vi "Launch Controller Actor.vi"(11 "RDS Root Actor in":refnum<class "RDS Root Actor.lvclass">) -> (3 "RDS Root Actor out":refnum<class "RDS Root Actor.lvclass">)   [LabVIEW 2015, in "RDS Root Actor.lvlib" / "RDS Root Actor.lvclass"]
uses:
  RDS Root Actor.lvclass
  Libraries/RDS Framework/RDS Message ID.ctl
  RDS Controller Actor/RDS Controller Actor/RDS Controller Actor/RDS Controller Actor.lvclass
  RDS Parent Actor/RDS Parent Actor/RDS Parent Actor.lvclass/RDS Parent Actor.ctl
  RDS Parent Actor/RDS Parent Actor/RDS Parent Actor.lvclass
  Libraries/RDS Child Messages/RDS Child Messages.lvlib
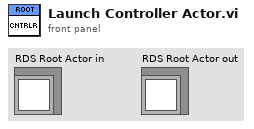
[diagram p1: front panel]
types:
  T1 = typedef "RDS Child Messages.lvlib/RDS Message ID.ctl" = enum16{"RDS Hello World", "String Message", "AIP_Status", "AIP_Command", "GPS_Data", "MCB_Command", "MCB_Status", "Compass_Data", "Depth_Data", "Battery_Data", "Contoller_State", "Set_Mag_Dev", "BTB_Shutdown", "State_Sample_Request", "State_Sample", "PID_Gains_Set", "Helm_Limiter_Set", "Helm_Heading_Command", "Helm_Steering_Command", "Helm_Status", "Controller_Message", "AIP_Set_Min_Depth", "Mission_Controller_State", "Mission_Upload", "Mission_Set_Op_and_Run", "Mission_Settings_Set"}
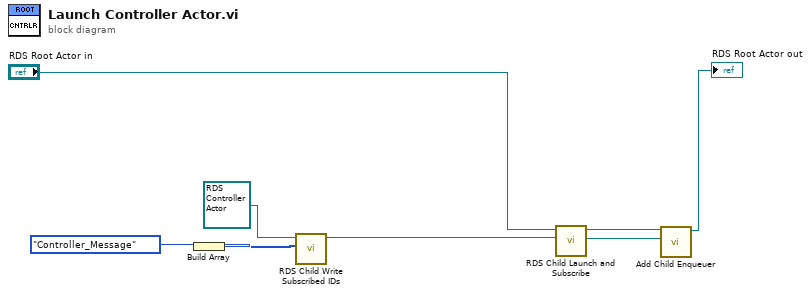
[diagram p0: block diagram]
diagram:
  n1 = Build Array(RDS_Message_ID."Controller_Message" ("RDS Message")) -> (w2:T1[])
  n2 = call "RDS Child Write Subscribed IDs.vi"("Subscribed IDs"=w2, "RDS Parent Actor in"=refnum<class "RDS Controller Actor.lvclass"> refnum ("RDS Controller Actor.lvlib:RDS Controller Actor.lvclass")) -> ("RDS Parent Actor out"=w5:refnum<class "RDS Controller Actor.lvclass">)  [unwired: 8 in, 1 out]
  n3 = call "RDS Child Launch and Subscribe.vi"("RDS Child in"=w5, "Caller Actor in"="RDS Root Actor in") -> ("Nested Actor's Enqueuer"=w7:refnum<class "Message Enqueuer.lvclass">, "Caller Actor Out"=w6:refnum<class "RDS Root Actor.lvclass">)  [unwired: 7 in, 1 out]
  n4 = call "Add Child Enqueuer.vi"("Nested Actor's Enqueuer"=w7, "RDS Root Actor in"=w6) -> ("RDS Root Actor out"=→"RDS Root Actor out":refnum<class "RDS Root Actor.lvclass">)  [unwired: 8 in, 1 out]
